vi "DUAL GAUGE-Conver4Int.vi"(0 "String in":string) -> (6 "ADC CH 1 out":u16, 8 "Integer2 out":u16, 10 "Integer3 out":u16, 15 "Integer4 out":u16)   [LabVIEW 2013, in "Dual Gauge.lvlib"]
uses:
  Dual Gauge.lvlib
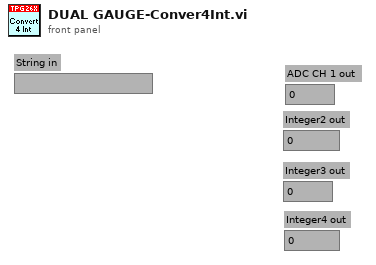
[diagram p1: front panel]
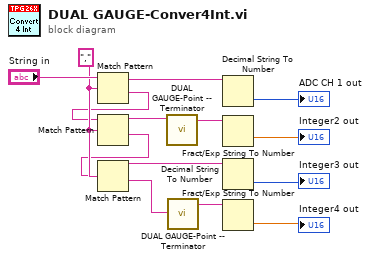
[diagram p0: block diagram]
diagram:
  w10 = "," ("regular expression")
  n1 = Match Pattern(string="String in", regular expression=w10) -> (before substring=w1:string, after substring=w6:string)  [unwired: 1 in, 2 out]
  n2 = Match Pattern(string=w6, regular expression=w10) -> (before substring=w11:string, after substring=w9:string)  [unwired: 1 in, 2 out]
  n3 = Match Pattern(string=w9, regular expression=w10) -> (before substring=w4:string, after substring=w3:string)  [unwired: 1 in, 2 out]
  n4 = call "DUAL GAUGE-Point -- Terminator.vi"("Eingangstring"=w11) -> ("Ausgangstring"=w8:string)
  n5 = call "DUAL GAUGE-Point -- Terminator.vi"("Eingangstring"=w3) -> ("Ausgangstring"=w7:string)
  n6 = Decimal String To Number(string=w1) -> (number=→"ADC CH 1 out":i32)  [unwired: 2 in, 1 out]
  n7 = Fract/Exp String To Number(string=w8) -> (number=→"Integer2 out":dbl)  [unwired: 3 in, 1 out]
  n8 = Decimal String To Number(string=w4) -> (number=→"Integer3 out":i32)  [unwired: 2 in, 1 out]
  n9 = Fract/Exp String To Number(string=w7) -> (number=→"Integer4 out":dbl)  [unwired: 3 in, 1 out]
